vi "常规五参数测量数据区.vi"(11 "数组":u16[](array[numeric]) format="%04xH") -> (3 "测量数据区":T1)   [LabVIEW 2016, in "斯坦道仪器.lvlib"]
panel:
  # "共占用26 WORD"
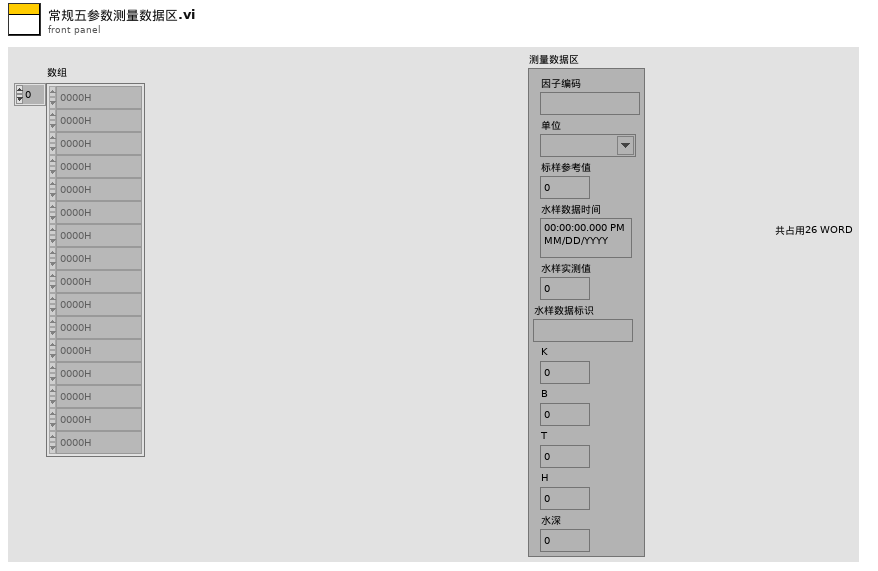
[diagram p1: front panel]
types:
  T1 = cluster{"因子编码":string, "单位":string, "标样参考值":sgl, "水样数据时间":timestamp, "水样实测值":sgl, "水样数据标识":string, "K":sgl, "B":sgl, "T":sgl, "H":sgl, "水深":sgl}
  T2 = cluster{string, string, "FLOAT":sgl, "time stamp":timestamp, "数值":sgl, "string":string, "FLOAT":sgl, "FLOAT":sgl, "FLOAT":sgl, "FLOAT":sgl, "FLOAT":sgl}
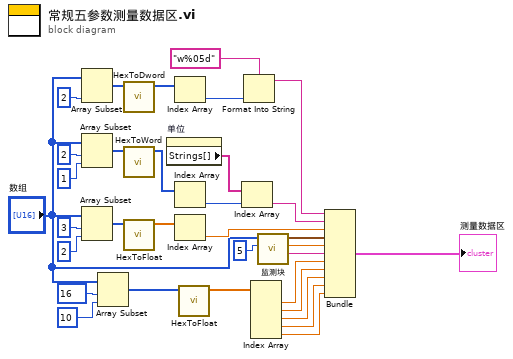
[diagram p0: block diagram]
diagram:
  n1 = Array Subset(array="数组", length=2 ("长度")) -> (w33:u16[])  [unwired: 1 in]
  n2 = Array Subset(array="数组", index=2 ("索引"), length=1 ("长度")) -> (w28:u16[])
  n3 = Array Subset(array="数组", index=3 ("索引"), length=2 ("长度")) -> (w24:u16[])
  n4 = Array Subset(array="数组", index=16 ("索引"), length=10 ("长度")) -> (w14:u16[])
  n5 = call "HexToDword.vi"("数组"=w33) -> ("DWORD"=w31:i32[])  [unwired: 10 in]
  n6 = call "HexToWord.vi"("数组"=w28) -> ("WORD"=w27:u16[])  [unwired: 10 in]
  n7 = call "HexToFloat.vi"("数组"=w24) -> ("FLOAT"=w23:sgl[])  [unwired: 10 in]
  n8 = property on="单位" class="CmbBox"() -> ("Strings[]"=w4:string[])  [unwired: 2 in, 2 out]
  n9 = Index Array(array=w31) -> (element=w2:i32)  [unwired: 1 in]
  n10 = Index Array(array=w27) -> (element=w6:u16)  [unwired: 1 in]
  n11 = Index Array(array=w23) -> (element=w22:sgl)  [unwired: 1 in]
  n12 = call "HexToFloat.vi"("数组"=w14) -> ("FLOAT"=w13:sgl[])  [unwired: 10 in]
  n13 = Index Array(array=w4, index=w6) -> (element=w5:string)
  n14 = Format Into String(format string="w%05d" ("格式字符串"), w2) -> (resulting string=w1:string)  [unwired: 2 in, 1 out]
  n15 = Index Array(array=w13) -> (element #1=w12:sgl, element #2=w11:sgl, element #3=w10:sgl, element #4=w9:sgl, element #5=w8:sgl)  [unwired: 5 in]
  n16 = call "监测块.vi"("索引"=5, "数组"="数组") -> ("string"=w19:string, "数值"=w20:sgl, "time stamp"=w21:timestamp)  [unwired: 7 in]
  n17 = Bundle(w1, w5, "FLOAT"=w22, "time stamp"=w21, "数值"=w20, "string"=w19, "FLOAT"=w12, "FLOAT"=w11, "FLOAT"=w10, "FLOAT"=w9, "FLOAT"=w8) -> (→"测量数据区":T2)  [unwired: 1 in]
